vi "Test Sweep Generate Waveforms.vi"(8 "error in (no error)":errorcluster, 11 "Generator in":refnum<class "Generator.lvclass">) -> (0 "error out":errorcluster, 3 "Generator in":refnum<class "Generator.lvclass">)   [LabVIEW 2019, in "Generator.lvclass"]
uses:
  Generator.lvclass
  typedefs/Generator.Sweep State--enum.ctl
  typedefs/AO.Channel.Function--Enum.ctl
  typedefs/AO.Channel--Cluster.ctl
  typedefs/Sweep.Pattern--Enum.ctl
  typedefs/Sweep.Channel--Cluster.ctl
  typedefs/Sweep.Channel--Cluster--Array.ctl
  typedefs/Sweep.Configuration--Cluster.ctl
  typedefs/AO.Channel--Cluster--Array.ctl
  typedefs/Sampling--Cluster.ctl
panel:
  in  "View initial wait?":bool=TRUE
  out "Intensity Graph":dbl[][](graph)
  out "sweep state out":T1
  in  "Sweep Pattern":cluster{"Channel":u16, "Sweep Pattern":dbl[]}[](array[cluster])=[{"Channel"=1, "Sweep Pattern"=[0.0, 0.0, 0.01, 0.01, -0.01, -0.01, 0.0, 0.0]}] {"Sweep Pattern" format="%#_3p"; "Channel" min=1 max=128}
  in  "milliseconds to wait":u32=145
  out "Updates":i32=49
  out "Waveform Graph":waveform(dbl)[](graph)
  in  "Configuration.Sweep":T2={"Sweep Time (s)"=5.0, "Initial Wait (s)"=2.0, "Return to Start"=FALSE, "Channels"=[{"Enable?"=TRUE, "Channel"=1, "Start"=0.0, "End"=0.1, "Pattern"=enum."Ramp /", "Table"=[]}]} {"Channels"."Table" format="%#_1f"; "Channels"."Channel" min=1 max=128; "Channels"."Start" format="%#_6p"; "Channels"."End" format="%#_6p"}
  in  "Sampling":T6
  in  "stop":bool
  in  "AO Channels":T7
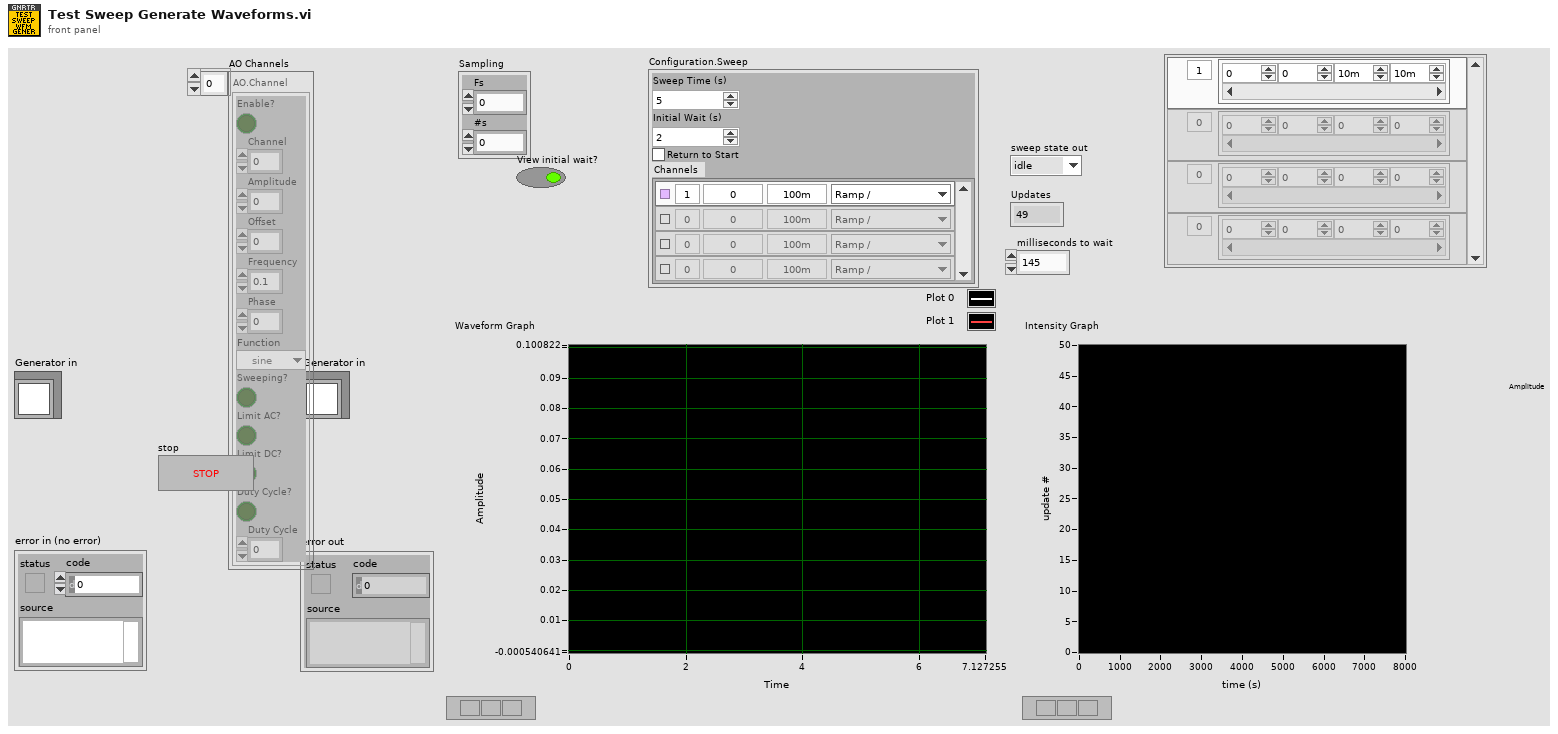
[diagram p1: front panel]
types:
  T1 = typedef "Generator.lvclass/Generator.Sweep State--enum.ctl" = enum16{"idle", "initialize", "wait", "sweep"}
  T2 = typedef "Generator.lvclass/Sweep.Configuration--Cluster.ctl" = cluster{"Sweep Time (s)":dbl, "Initial Wait (s)":dbl, "Return to Start":bool, "Channels":T3}
  T3 = typedef "Generator.lvclass/Sweep.Channel--Cluster--Array.ctl" = T4[]
  T4 = typedef "Generator.lvclass/Sweep.Channel--Cluster.ctl" = cluster{"Enable?":bool, "Channel":u16, "Start":dbl, "End":dbl, "Pattern":T5, "Table":dbl[]}
  T5 = typedef "Generator.lvclass/Sweep.Pattern--Enum.ctl" = enum16{"Ramp /", "Ramp /\\", "Smooth Ramp _/", "Smooth Ramp _/\\_", "Table"}
  T6 = typedef "Generator.lvclass/Sampling--Cluster.ctl" = cluster{"Fs":dbl, "#s":dbl}
  T7 = typedef "Generator.lvclass/AO.Channel--Cluster--Array.ctl" = T8[]
  T8 = typedef "Generator.lvclass/AO.Channel--Cluster.ctl" = cluster{"Enable?":bool, "Channel":i32, "Amplitude":dbl, "Offset":dbl, "Frequency":dbl, "Phase":dbl, "Function":T9, "Sweeping?":bool, "Limit AC?":bool, "Limit DC?":bool, "Duty Cycle?":bool, "Duty Cycle":dbl}
  T9 = typedef "Generator.lvclass/AO.Channel.Function--Enum.ctl" = enum16{"sine", "square", "triangle", "saw"}
  T10 = typedef "Generator.lvclass/Waveforms--Cluster.ctl" = cluster{"AO":waveform(dbl)[], "REF_X":waveform(dbl)[], "REF_Y":waveform(dbl)[]}
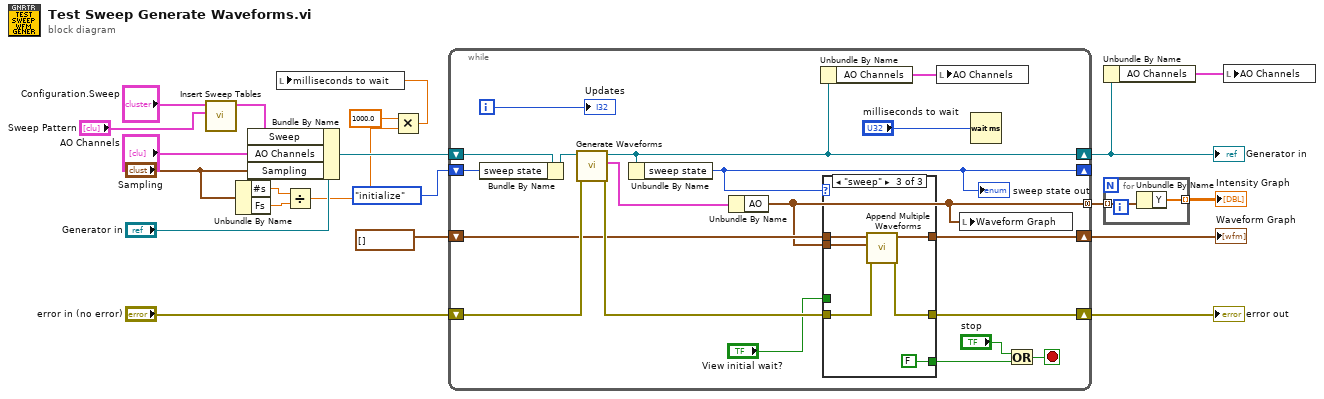
[diagram p0: block diagram]
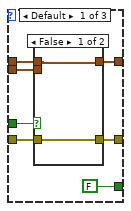
[diagram p2: hidden frame]
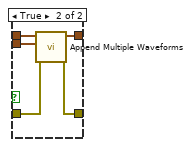
[diagram p3: hidden frame]
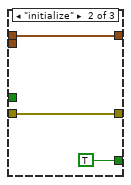
[diagram p4: hidden frame]
diagram:
  n1 = call "Insert Sweep Tables.vi"("Channels New"="Sweep Pattern", "Sweep Configuration in"="Configuration.Sweep") -> ("Sweep Configuration out"=w17:T2)  [unwired: 9 in]
  n2 = Unbundle By Name("Sampling") -> ("#s"=w5:dbl, "Fs"=w4:dbl)
  n3 = Bundle By Name(cluster="Generator in", "Sweep"=w17, "AO Channels"="AO Channels", "Sampling"="Sampling") -> (w12:refnum<class "Generator.lvclass">)
  n4 = Divide(x=w5, y=w4) -> (x/y=w3:dbl)
  n5 = Multiply(x=1000.0, y=w3) -> (x*y=w1:dbl)
  n6 = local write "milliseconds to wait"(w1) -> ()
  n7 = while {
    shift-right: [w39] -> w21
    shift-left: "error in (no error)" -> [w40]
    shift-right: [w24] -> w14
    shift-left: w12 -> [w27]
    shift-right: [w33] -> w9
    shift-left: waveform(dbl)[] [] ("Waveform out []") -> [w34]
    tunnel: [w30] -> w8 mode=concatenating
    shift-right: [w22] -> _
    shift-left: Generator.Sweep_State--enum."initialize" ("sweep state") -> [w26]
    i -> [w38]
    stop <- w37 stop-if-true
    n8 = Bundle By Name(cluster=w27, "sweep state"=w26) -> (w25:refnum<class "Generator.lvclass">)
    n9 = call "Generate Waveforms.vi"("error in (no error)"=w40, "Generator.lvclass"=w25) -> ("error out"=w35:errorcluster, "Waveforms out"=w23:T10, "Generator.lvclass"=w24:refnum<class "Generator.lvclass">)  [unwired: 6 in, 1 out]
    n10 = Unbundle By Name(w24) -> ("sweep state"=w22:T1)
    "sweep state out" <- w22
    n11 = Unbundle By Name(w23) -> ("AO"=w30:waveform(dbl)[])
    n12 = Unbundle By Name(w24) -> ("AO Channels"=w36:T7)
    n13 = case shown="\"sweep\"" w22 {
      tunnel: [w43 w56 w63] -> w39
      tunnel: w35 -> [w42 w56 w62]
      tunnel: w30 -> [w46 _ w61]
      tunnel: w34 -> [w44 w57 w60]
      tunnel: [w45 w57 w59] -> w33
      tunnel: [FALSE TRUE FALSE] -> w31
      tunnel: "View initial wait?" -> [w41 _ _]
      frame Default {
        n14 = case shown="False" w41 {
          tunnel: w46 -> [_ w54]
          tunnel: [w49 w53] -> w45
          tunnel: w44 -> [w49 w52]
          tunnel: [w48 w51] -> w43
          tunnel: w42 -> [w48 w50]
          frame False {
          }
          frame True {
            n15 = call "Append Multiple Waveforms.vi"("error in (no error)"=w50, "Waveform B []"=w54, "Waveforrm A []"=w52) -> ("error out"=w51:errorcluster, "Waveform out []"=w53:waveform(dbl)[])  [unwired: 7 in]
          }
        }
      }
      frame "initialize" {
      }
      frame "sweep" {
        n16 = call "Append Multiple Waveforms.vi"("error in (no error)"=w62, "Waveform B []"=w61, "Waveforrm A []"=w60) -> ("error out"=w63:errorcluster, "Waveform out []"=w59:waveform(dbl)[])  [unwired: 7 in]
      }
    }
    n17 = local write "AO Channels"(w36) -> ()
    n18 = local write "Waveform Graph"(w30) -> ()
    n19 = Wait (ms)(milliseconds to wait="milliseconds to wait") -> ()  [unwired: 1 out]
    n20 = Or(x="stop", y=w31) -> (x .or. y?=w37:bool)
    "Updates" <- w38
  }
  "error out" <- w21
  "Generator in" <- w14
  "Waveform Graph" <- w9
  n21 = Unbundle By Name(w14) -> ("AO Channels"=w15:T7)
  n22 = for {
    tunnel: w8 -> [w65] mode=indexing
    tunnel: [w64] -> w7 mode=indexing
    n23 = Unbundle By Name(w65) -> ("Y"=w64:dbl[])
  }
  "Intensity Graph" <- w7
  n24 = local write "AO Channels"(w15) -> ()
